vi "ClimberSystem.vi"(8 "Reset Climb Encoder":bool, 11 "Desired Angle (deg)":dbl) -> ()   [LabVIEW 2018]
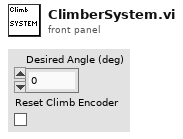
[diagram p1: front panel]
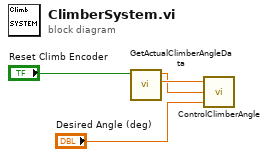
[diagram p0: block diagram]
diagram:
  n1 = call "GetActualClimberAngleData.vi"("Reset Encoder"="Reset Climb Encoder") -> ("Encoder Speed (deg/s)"=w3:dbl, "Encoder Angle (deg)"=w1:dbl)  [unwired: 9 in]
  n2 = call "ControlClimberAngle.vi"("Goal Angle (deg)"="Desired Angle (deg)", "Climber Angle (deg)"=w1, "Angular Velocity (deg/s)"=w3) -> ()  [unwired: 1 in]
